vi "WRTxt.vi"(8 "error in":errorcluster caption="错误输入", 9 "Text":string, 11 "FilePath":path) -> (0 "error out":errorcluster caption="错误输出")   [LabVIEW 2013]
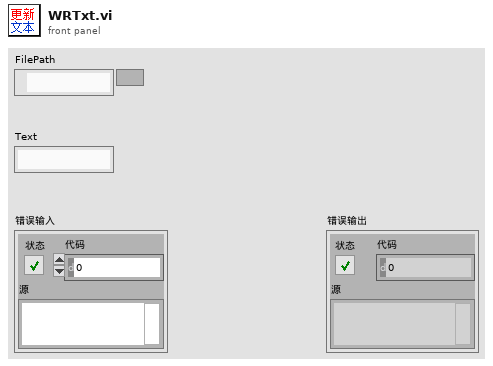
[diagram p1: front panel]
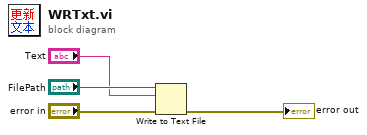
[diagram p0: block diagram]
diagram:
  n1 = Write to Text File(file (use dialog)="FilePath", text="Text", error in="error in") -> (error out=→"error out":errorcluster)  [unwired: 1 in, 2 out]
